vi "uxx-u8s.vi"   [LabVIEW 2012]
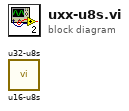
[diagram p0: block diagram]
diagram:
  n1 = call "u16-u8s.vi"() -> ()  [unwired: 11 in, 1 out]
  n2 = call "u32-u8s.vi"() -> ()  [unwired: 11 in, 1 out]
